vi "Actual Sample Rate.vi"(8 "error in (no error)":errorcluster {"code" format="%.0x"}, 11 "VISA Resource Name":refnum<visa-resource-name>) -> (0 "error out":errorcluster {"code" format="%.0x"}, 2 "Sample Rate":dbl format="%.2p", 3 "VISA Resource Name Out":refnum<visa-resource-name>)   [LabVIEW 2010, in "Tektronix TDS 3000 Series.lvlib"]
doc: "Returns the current sample rate of the osilloscope."
uses:
  <instrlib>/Tektronix TDS 3000 Series/Tektronix TDS 3000 Series.lvlib
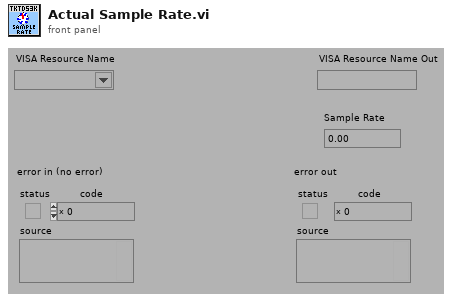
[diagram p1: front panel]
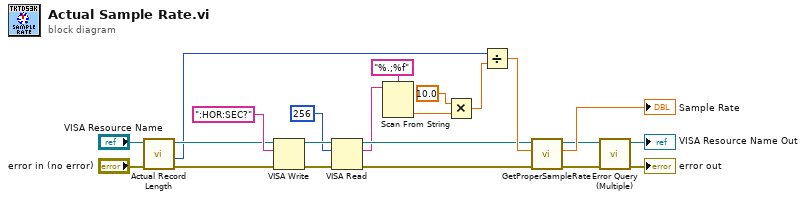
[diagram p0: block diagram]
diagram:
  n1 = call <instrlib>:"Actual Record Length.vi"("error in (no error)"="error in (no error)", "VISA Resource Name"="VISA Resource Name") -> ("error out"=w16:errorcluster, "Actual Record Length"=w12:i32, "VISA Resource Name Out"=w17:refnum<visa-resource-name>)  [unwired: 7 in]
  n2 = VISA Write(VISA resource name=w17, write buffer=":HOR:SEC?", error in (no error)=w16) -> (VISA resource name out=w22:refnum<visa-resource-name>, error out=w21:errorcluster)  [unwired: 1 out]
  n3 = VISA Read(VISA resource name=w22, byte count=u32 256, error in (no error)=w21) -> (VISA resource name out=w10:refnum<visa-resource-name>, read buffer=w6:string, error out=w9:errorcluster)  [unwired: 1 out]
  n4 = Scan From String(format string="%.;%f", input string=w6) -> (output 1=w5:dbl)  [unwired: 3 in, 3 out]
  n5 = Multiply(x=10.0, y=w5) -> (x*y=w13:dbl)
  n6 = Divide(x=w12, y=w13) -> (x/y=w11:dbl)
  n7 = call <instrlib>:"GetProperSampleRate.vi"("error in (no error)"=w9, "Sample Rate (0.00)"=w11, "VISA Resource Name"=w10) -> ("error out"=w3:errorcluster, "New Sample Rate"=→"Sample Rate":dbl, "VISA Resource Name Out"=w4:refnum<visa-resource-name>)  [unwired: 6 in]
  n8 = call <instrlib>:"Error Query (Multiple).vi"("error in (no error)"=w3, "VISA Resource Name"=w4) -> ("error out"=→"error out":errorcluster, "VISA Resource Name Out"=→"VISA Resource Name Out":refnum<visa-resource-name>)  [unwired: 6 in, 2 out]
